vi "Data-120127-TF_20-HP_3_Analyze.vi"() -> ()   [LabVIEW 2011]
uses:
  <vilib>/Utility/file.llb/Write To Spreadsheet File (I64).vi
  <vilib>/Analysis/NI_AALPro.lvlib
panel:
  out "x/y":dbl[](array[numeric])
  in  "LUT filename":string
  in  "save LUT":bool
  in  "stop":bool
  in  "balance parameter":dbl=-1.0
  out "Obtained LUT":cluster{"LevelsToCharacterize":i16[], i32[]}(graph)
  in  "start index (0)":i32
  in  "length2":i32
  in  "length1":i32
  out "Phase calculated \nfrom power in 1:st order":T1(graph)
  in  "LevelsToCharacterize":i16[](array[numeric])=[0, 1, 2, 3, 4, 5, 6, 7, 8, 9, 10, 11, 12, 13, 14, 15, 16, 17, 18, 19, 20, 21, 22, 23, 24, 25, 26, 27, 28, 29, 30, 31, 32, 33, 34, 35, 36, 37, 38, 39, 40, 41, 42, 43, 44, 45, 46, 47, 48, 49, 50, 51, 52, 53, 54, 55, 56, 57, 58, 59, 60, 61, 62, 63, 64, 65, 66, 67, 68, 69, 70, 71, 72, 73, 74, 75, 76, 77, 78, 79, 80, 81, 82, 83, 84, 85, 86, 87, 88, 89, 90, 91, 92, 93, 94, 95, 96, 97, 98, 99, 100, 101, 102, 103, 104, 105, 106, 107, 108, 109, 110, 111, 112, 113, 114, 115, 116, 117, 118, 119, 120, 121, 122, 123, 124, 125, 126, 128, 129, 130, 131, 132, 133, 134, 135, 136, 137, 138, 139, 140, 141, 142, 143, 144, 145, 146, 147, 148, 149, 150, 151, 152, 153, 154, 155, 156, 157, 158, 159, 160, 161, 162, 163, 164, 165, 166, 167, 168, 169, 170, 171, 172, 173, 174, 175, 176, 177, 178, 179, 180, 181, 182, 183, 184, 185, 186, 187, 188, 189, 190, 191, 192, 193, 194, 195, 196, 197, 198, 199, 200, 201, 202, 203, 204, 205, 206, 207, 208, 209, 210, 211, 212, 213, 214, 215, 216, 217, 218, 219, 220, 221, 222, 223, 224, 225, 226, 227, 228, 229, 230, 231, 232, 233, 234, 235, 236, 237, 238, 239, 240, 241, 242, 243, 244, 245, 246, 247, 248, 249, 250, 251, 252, 253, 254, 255]
  in  "NormalizedPowerInROI":dbl[](array[numeric])=[-0.0012623561127990072, -0.0009949077838161667, 0.0013158457785955753, -0.00022465659634558603, 0.0011660747143651846, 0.001155376781205871, -0.0002460524626642133, 0.0015405023749411615, 0.0004172193932132312, -0.0012837519791176345, 0.0019577217681543925, 0.0026423894903504644, 0.0016795755060122384, 0.0006097821900808764, -0.0005883863237622491, -0.0013586375112328297, 0.0004600111258504857, 0.0014121271770293979, -0.001155376781205871, 6.418759895588172e-05, 0.00014977106423039069, 0.0008558346527450896, 0.00040652146005391756, -8.558346527450897e-05, 0.0013586375112328297, 0.0010376995164534213, 0.002171680431340665, 0.002021909367110274, 0.001947023834995079, 0.0019363259018357654, 0.003658693140485258, 0.003412640677821045, 0.005627112841798965, 0.006718302024048954, 0.00632247849715435, 0.008579742393769524, 0.011339809148872438, 0.015105481620950833, 0.014570584962985151, 0.018486028499293938, 0.025150840857546323, 0.02946210792074971, 0.03368779151867859, 0.045348538662330434, 0.05791861012452394, 0.07316316487654585, 0.09602464803799905, 0.11769866061876845, 0.14657238221575591, 0.19568659335016475, 0.23480893491377466, 0.28100261029569085, 0.34906286105524414, 0.42603449013650563, 0.4959668791989388, 0.5669155719115067, 0.6520497239933245, 0.7287753006119218, 0.8019491634216269, 0.8597180024819205, 0.9141062946638709, 0.9605567204416107, 0.9904360477555736, 1.0, 0.9995399888741495, 0.9942445119602893, 0.9689439000385126, 0.9349886601908511, 0.8950853695066113, 0.8518657195429843, 0.8007509949077838, 0.7483739141597844, 0.6922097650733878, 0.6373400658992683, 0.5830694509820703, 0.5282532414737473, 0.4721104882536694, 0.41934828191193463, 0.3675595874876974, 0.3181779280243057, 0.27067910479695323, 0.22638966151739484, 0.18594077624203004, 0.1496212931661603, 0.11472463520047926, 0.08802259403483247, 0.061545209465531256, 0.039871196884761866, 0.023321494287303693, 0.010013265437117549, 0.00197911763447302, -0.0005135007916470538, -0.002952629551970559, 0.0011981685138431255, 0.008708117591681287, 0.021684710513928708, 0.035891565749497194, 0.05534040823312936, 0.07456459412041594, 0.09704095168813386, 0.12340065899268261, 0.1529911421113441, 0.18239976036629724, 0.21186186828704695, 0.24633060892635542, 0.2787453463990757, 0.3126684924472592, 0.34639907569857503, 0.3789528863023664, 0.41143181137404256, 0.4440177157773118, 0.4763575677179169, 0.5088150969232744, 0.540384697676409, 0.5673434892378793, 0.5935641234113569, 0.623924857717489, 0.6465830801489152, 0.6633467414095596, 0.6817899781762163, 0.6978689717146648, 0.7188690145063974, 0.7443193974924045, 0.7629124053232915, 0.7772476357567718, 0.7886730283709188, 0.8057255338268646, 0.8260943985621978, 0.8331015447815482, 0.8469553682228593, 0.8563802473362147, 0.8585947195001926, 0.8620501519106508, 0.8718280628182635, 0.8698382472506312, 0.8843553425478198, 0.8859172407890795, 0.8949783901750182, 0.9026167144507681, 0.9010869100089862, 0.9017394839317044, 0.909944798664898, 0.9097629338011896, 0.9119667080320082, 0.9129402199495058, 0.9127904488852754, 0.9096666524027558, 0.909538277204844, 0.9148658479181823, 0.9178077795369934, 0.9157751722367239, 0.9149086396508195, 0.9118062390346185, 0.9108541229834396, 0.9092494330095425, 0.9067354187171038, 0.9023599640549446, 0.8996212931661604, 0.8960802772904275, 0.8940904617227952, 0.8880033377551457, 0.885692584192734, 0.8871154093029227, 0.8832320595660919, 0.8782789165133297, 0.8721490008130429, 0.8698810389832684, 0.8658372202490479, 0.8665860755701998, 0.8630878514271043, 0.862670632033891, 0.8588514698960161, 0.8548611408275921, 0.8515661774145236, 0.8419487355043006, 0.8395523984766143, 0.834085754632205, 0.8324489708588301, 0.8262976592922248, 0.8256771791689845, 0.8217082459668792, 0.8199002952629552, 0.8189695750780949, 0.8101972698874578, 0.806281826351149, 0.803179425734948, 0.7962899567803501, 0.791069365398605, 0.7887907056356712, 0.7833454576575806, 0.7815802986862939, 0.7748085069964483, 0.7704651461337669, 0.7716740125807694, 0.7659506183405366, 0.7642603449013651, 0.7584192733963798, 0.7521395866318628, 0.7504065214600539, 0.7488446232187941, 0.7458919936668236, 0.7393983482391202, 0.7325302751508409, 0.7318028156960076, 0.7264431511831914, 0.725202190936711, 0.7229556249732552, 0.7171359493345886, 0.7149856647695665, 0.7110595233000985, 0.7051970559287946, 0.7019341863152039, 0.6973019812572211, 0.6958042706149172, 0.6908190337626771, 0.6868180067610937, 0.6857589113783217, 0.6839723565407163, 0.6755851769438145, 0.6782382643673243, 0.6737130386409346, 0.6685887286576233, 0.6641062946638709, 0.6594954854722068, 0.6587038384184175, 0.6567675125165818, 0.6524562454533784, 0.6494501262356113, 0.6455667764987805, 0.645823526894604, 0.6404317685823099, 0.6408061962428859, 0.6373721596987462, 0.6372758783003124, 0.6357246779922119, 0.6355321151953442, 0.6345158115452094, 0.6297659292224742, 0.6274765715263811, 0.6265993410073174, 0.6249732551671017, 0.6257969960203689, 0.6232936796610895, 0.6268026017373444, 0.6240104411827635, 0.6218173648851042, 0.6150455731952587, 0.6176130771534939, 0.6134729770208396, 0.6122748085069964, 0.6091082202918396, 0.6113440883221362, 0.6081775001069794, 0.6035987847147931, 0.603866233043776]
  out "Power in ROI vs\nGrating Levels\nTo Characterize":T2(graph)
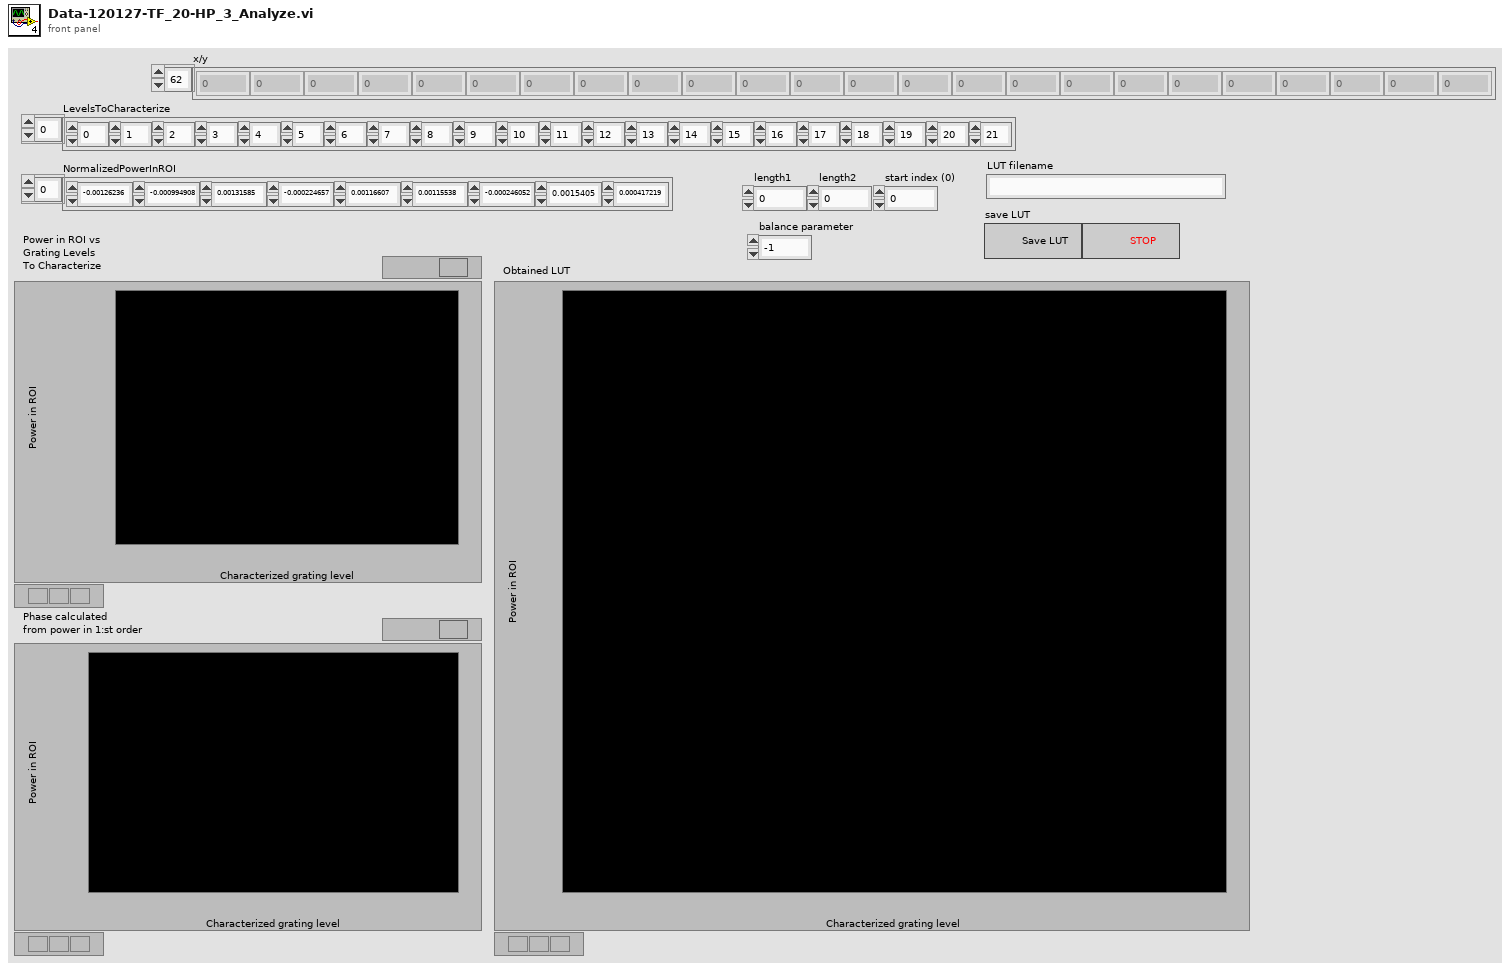
[diagram p1: front panel]
types:
  T1 = cluster{"LevelsToCharacterize":i16[], "NormalizedPowerInROI":dbl[]}
  T2 = cluster{"LevelsToCharacterize":i16[], "Best Cubic Spline Fit":dbl[]}[]
  T3 = cluster{"LevelsToCharacterize":i16[], "Best Cubic Spline Fit":dbl[]}
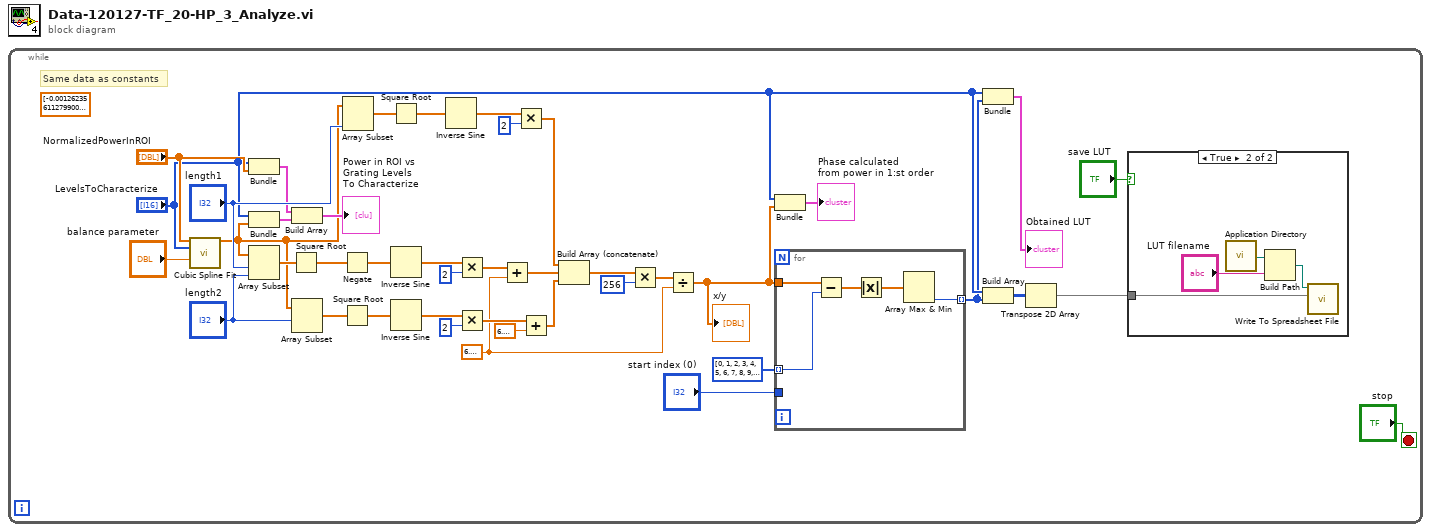
[diagram p0: block diagram]
diagram:
  n1 = while {
    stop <- "stop" stop-if-true
    w17 = 6.283185307179586
    (unwired) dbl[] [-0.0012623561127990072, -0.0009949077838161667, 0.0013158457785955753, -0.00022465659634558603, 0.0011660747143651846, 0.001155376781205871, -0.0002460524626642133, 0.0015405023749411615, 0.0004172193932132312, -0.0012837519791176345, 0.0019577217681543925, 0.0026423894903504644, 0.0016795755060122384, 0.0006097821900808764, -0.0005883863237622491, -0.0013586375112328297, 0.0004600111258504857, 0.0014121271770293979, -0.001155376781205871, 6.418759895588172e-05, 0.00014977106423039069, 0.0008558346527450896, 0.00040652146005391756, -8.558346527450897e-05, 0.0013586375112328297, 0.0010376995164534213, 0.002171680431340665, 0.002021909367110274, 0.001947023834995079, 0.0019363259018357654, 0.003658693140485258, 0.003412640677821045, 0.005627112841798965, 0.006718302024048954, 0.00632247849715435, 0.008579742393769524, 0.011339809148872438, 0.015105481620950833, 0.014570584962985151, 0.018486028499293938, 0.025150840857546323, 0.02946210792074971, 0.03368779151867859, 0.045348538662330434, 0.05791861012452394, 0.07316316487654585, 0.09602464803799905, 0.11769866061876845, 0.14657238221575591, 0.19568659335016475, 0.23480893491377466, 0.28100261029569085, 0.34906286105524414, 0.42603449013650563, 0.4959668791989388, 0.5669155719115067, 0.6520497239933245, 0.7287753006119218, 0.8019491634216269, 0.8597180024819205, 0.9141062946638709, 0.9605567204416107, 0.9904360477555736, 1.0, 0.9995399888741495, 0.9942445119602893, 0.9689439000385126, 0.9349886601908511, 0.8950853695066113, 0.8518657195429843, 0.8007509949077838, 0.7483739141597844, 0.6922097650733878, 0.6373400658992683, 0.5830694509820703, 0.5282532414737473, 0.4721104882536694, 0.41934828191193463, 0.3675595874876974, 0.3181779280243057, 0.27067910479695323, 0.22638966151739484, 0.18594077624203004, 0.1496212931661603, 0.11472463520047926, 0.08802259403483247, 0.061545209465531256, 0.039871196884761866, 0.023321494287303693, 0.010013265437117549, 0.00197911763447302, -0.0005135007916470538, -0.002952629551970559, 0.0011981685138431255, 0.008708117591681287, 0.021684710513928708, 0.035891565749497194, 0.05534040823312936, 0.07456459412041594, 0.09704095168813386, 0.12340065899268261, 0.1529911421113441, 0.18239976036629724, 0.21186186828704695, 0.24633060892635542, 0.2787453463990757, 0.3126684924472592, 0.34639907569857503, 0.3789528863023664, 0.41143181137404256, 0.4440177157773118, 0.4763575677179169, 0.5088150969232744, 0.540384697676409, 0.5673434892378793, 0.5935641234113569, 0.623924857717489, 0.6465830801489152, 0.6633467414095596, 0.6817899781762163, 0.6978689717146648, 0.7188690145063974, 0.7443193974924045, 0.7629124053232915, 0.7772476357567718, 0.7886730283709188, 0.8057255338268646, 0.8260943985621978, 0.8331015447815482, 0.8469553682228593, 0.8563802473362147, 0.8585947195001926, 0.8620501519106508, 0.8718280628182635, 0.8698382472506312, 0.8843553425478198, 0.8859172407890795, 0.8949783901750182, 0.9026167144507681, 0.9010869100089862, 0.9017394839317044, 0.909944798664898, 0.9097629338011896, 0.9119667080320082, 0.9129402199495058, 0.9127904488852754, 0.9096666524027558, 0.909538277204844, 0.9148658479181823, 0.9178077795369934, 0.9157751722367239, 0.9149086396508195, 0.9118062390346185, 0.9108541229834396, 0.9092494330095425, 0.9067354187171038, 0.9023599640549446, 0.8996212931661604, 0.8960802772904275, 0.8940904617227952, 0.8880033377551457, 0.885692584192734, 0.8871154093029227, 0.8832320595660919, 0.8782789165133297, 0.8721490008130429, 0.8698810389832684, 0.8658372202490479, 0.8665860755701998, 0.8630878514271043, 0.862670632033891, 0.8588514698960161, 0.8548611408275921, 0.8515661774145236, 0.8419487355043006, 0.8395523984766143, 0.834085754632205, 0.8324489708588301, 0.8262976592922248, 0.8256771791689845, 0.8217082459668792, 0.8199002952629552, 0.8189695750780949, 0.8101972698874578, 0.806281826351149, 0.803179425734948, 0.7962899567803501, 0.791069365398605, 0.7887907056356712, 0.7833454576575806, 0.7815802986862939, 0.7748085069964483, 0.7704651461337669, 0.7716740125807694, 0.7659506183405366, 0.7642603449013651, 0.7584192733963798, 0.7521395866318628, 0.7504065214600539, 0.7488446232187941, 0.7458919936668236, 0.7393983482391202, 0.7325302751508409, 0.7318028156960076, 0.7264431511831914, 0.725202190936711, 0.7229556249732552, 0.7171359493345886, 0.7149856647695665, 0.7110595233000985, 0.7051970559287946, 0.7019341863152039, 0.6973019812572211, 0.6958042706149172, 0.6908190337626771, 0.6868180067610937, 0.6857589113783217, 0.6839723565407163, 0.6755851769438145, 0.6782382643673243, 0.6737130386409346, 0.6685887286576233, 0.6641062946638709, 0.6594954854722068, 0.6587038384184175, 0.6567675125165818, 0.6524562454533784, 0.6494501262356113, 0.6455667764987805, 0.645823526894604, 0.6404317685823099, 0.6408061962428859, 0.6373721596987462, 0.6372758783003124, 0.6357246779922119, 0.6355321151953442, 0.6345158115452094, 0.6297659292224742, 0.6274765715263811, 0.6265993410073174, 0.6249732551671017, 0.6257969960203689, 0.6232936796610895, 0.6268026017373444, 0.6240104411827635, 0.6218173648851042, 0.6150455731952587, 0.6176130771534939, 0.6134729770208396, 0.6122748085069964, 0.6091082202918396, 0.6113440883221362, 0.6081775001069794, 0.6035987847147931, 0.603866233043776] ("NormalizedPowerInROI 2")
    # "Same data as constants"
    n2 = call <vilib>:"Cubic Spline Fit.vi"("Y"="NormalizedPowerInROI", "X"="LevelsToCharacterize", "balance parameter"="balance parameter") -> ("Best Cubic Spline Fit"=w8:dbl[])  [unwired: 11 in, 1 out]
    n3 = Bundle("LevelsToCharacterize"="LevelsToCharacterize", "NormalizedPowerInROI"="NormalizedPowerInROI") -> (w12:T1)  [unwired: 1 in]
    n4 = Bundle("LevelsToCharacterize"="LevelsToCharacterize", "Best Cubic Spline Fit"=w8) -> (w11:T3)  [unwired: 1 in]
    n5 = Array Subset(array=w8, index="length1", length="length2") -> (w33:dbl[])
    n6 = Square Root(x=w33) -> (sqrt(x)=w35:dbl[])
    n7 = Build Array(w12, w11) -> (→"Power in ROI vs\nGrating Levels\nTo Characterize":T2)
    n8 = Array Subset(array=w8, index="length2") -> (w25:dbl[])  [unwired: 1 in]
    n9 = Negate(x=w35) -> (-x=w32:dbl[])
    n10 = Square Root(x=w25) -> (sqrt(x)=w24:dbl[])
    n11 = Array Subset(array=w8, length="length1") -> (w37:dbl[])  [unwired: 1 in]
    n12 = Square Root(x=w37) -> (sqrt(x)=w40:dbl[])
    n13 = Inverse Sine(1:w32) -> (0:w34:dbl[])
    n14 = Inverse Sine(1:w24) -> (0:w28:dbl[])
    n15 = Inverse Sine(1:w40) -> (0:w41:dbl[])
    n16 = Multiply(x=w34, y=2 ("Sum")) -> (x*y=w31:dbl[])
    n17 = Multiply(x=w28, y=2 ("Sum")) -> (x*y=w23:dbl[])
    n18 = Add(x=w31, y=w17) -> (x+y=w29:dbl[])
    n19 = Multiply(x=w41, y=2 ("Sum")) -> (x*y=w30:dbl[])
    n20 = Add(x=w23, y=6.283185307179586) -> (x+y=w22:dbl[])
    n21 = Build Array (concatenate)(w30, w29, w22) -> (w20:dbl[])
    n22 = Multiply(x=w20, y=256) -> (x*y=w18:dbl[])
    n23 = Divide(x=w18, y=w17) -> (x/y=w15:dbl[])
    "x/y" <- w15
    n24 = Bundle("LevelsToCharacterize"="LevelsToCharacterize", w15) -> (→"Phase calculated \nfrom power in 1:st order":cluster{"LevelsToCharacterize":i16[], dbl[]})  [unwired: 1 in]
    n25 = for {
      tunnel: i16[] [0, 1, 2, 3, 4, 5, 6, 7, 8, 9, 10, 11, 12, 13, 14, 15, 16, 17, 18, 19, 20, 21, 22, 23, 24, 25, 26, 27, 28, 29, 30, 31, 32, 33, 34, 35, 36, 37, 38, 39, 40, 41, 42, 43, 44, 45, 46, 47, 48, 49, 50, 51, 52, 53, 54, 55, 56, 57, 58, 59, 60, 61, 62, 63, 64, 65, 66, 67, 68, 69, 70, 71, 72, 73, 74, 75, 76, 77, 78, 79, 80, 81, 82, 83, 84, 85, 86, 87, 88, 89, 90, 91, 92, 93, 94, 95, 96, 97, 98, 99, 100, 101, 102, 103, 104, 105, 106, 107, 108, 109, 110, 111, 112, 113, 114, 115, 116, 117, 118, 119, 120, 121, 122, 123, 124, 125, 126, 128, 129, 130, 131, 132, 133, 134, 135, 136, 137, 138, 139, 140, 141, 142, 143, 144, 145, 146, 147, 148, 149, 150, 151, 152, 153, 154, 155, 156, 157, 158, 159, 160, 161, 162, 163, 164, 165, 166, 167, 168, 169, 170, 171, 172, 173, 174, 175, 176, 177, 178, 179, 180, 181, 182, 183, 184, 185, 186, 187, 188, 189, 190, 191, 192, 193, 194, 195, 196, 197, 198, 199, 200, 201, 202, 203, 204, 205, 206, 207, 208, 209, 210, 211, 212, 213, 214, 215, 216, 217, 218, 219, 220, 221, 222, 223, 224, 225, 226, 227, 228, 229, 230, 231, 232, 233, 234, 235, 236, 237, 238, 239, 240, 241, 242, 243, 244, 245, 246, 247, 248, 249, 250, 251, 252, 253, 254, 255] ("LevelsToCharacterize 2") -> [w51] mode=indexing
      tunnel: "start index (0)" -> [_]
      tunnel: w15 -> [w48]
      tunnel: [w47] -> w4 mode=indexing
      n26 = Subtract(x=w48, y=w51) -> (x-y=w50:dbl[])
      n27 = Absolute Value(x=w50) -> (abs(x)=w49:dbl[])
      n28 = Array Max & Min(array=w49) -> (min index (indices)=w47:i32)  [unwired: 3 out]
    }
    n29 = Bundle("LevelsToCharacterize"="LevelsToCharacterize", w4) -> (→"Obtained LUT":cluster{"LevelsToCharacterize":i16[], i32[]})  [unwired: 1 in]
    n30 = Build Array("LevelsToCharacterize", w4) -> (w3:i32[][])
    n31 = Transpose 2D Array(2D array=w3) -> (transposed array=w1:i32[][])
    n32 = case shown="True" "save LUT" {
      tunnel: w1 -> [_ w43]
      frame False {
      }
      frame True {
        n33 = call <vilib>:"Application Directory.vi"() -> ("Application Directory"=w46:path)
        n34 = Build Path(base path=w46, name or relative path="LUT filename") -> (appended path=w45:path)
        n35 = call-poly <vilib>:"Write To Spreadsheet File.vi"("2D data"=w43, "file path (dialog if empty)"=w45) -> ()  [unwired: 6 in, 1 out]
      }
    }
  }
